vi "StringSplitter.vi"(1 "Input String":string="FPSP0RP0FS0TL0PP50%TD1000FEBL1CL0RL1FL0AL1HL1G3") -> (14 "S0":string, 15 "S1":string, 16 "S2":string, 17 "S3":string, 18 "S4":string, 19 "S5":string)   [LabVIEW 2014]
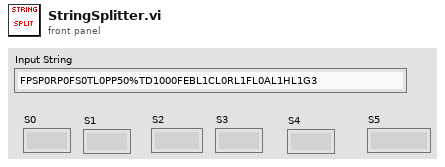
[diagram p1: front panel]
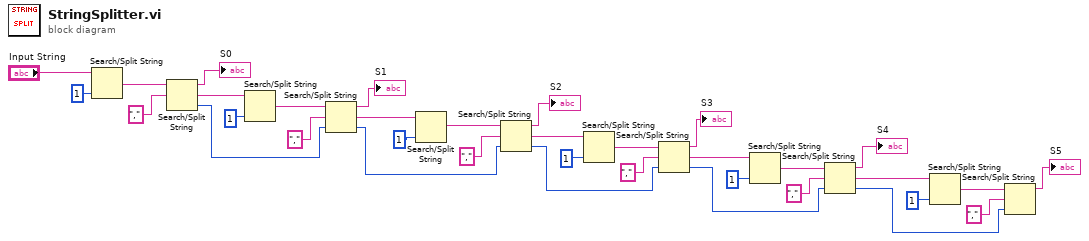
[diagram p0: block diagram]
diagram:
  n1 = Search/Split String(string="Input String", offset (0)=1) -> (match + rest of string=w33:string)  [unwired: 1 in, 2 out]
  n2 = Search/Split String(string=w33, search string/char (-)=",") -> (substring before match=→"S0":string, match + rest of string=w30:string, offset of match=w26:i32)  [unwired: 1 in]
  n3 = Search/Split String(string=w30, offset (0)=1) -> (match + rest of string=w28:string)  [unwired: 1 in, 2 out]
  n4 = Search/Split String(string=w28, search string/char (-)=",", offset (0)=w26) -> (substring before match=→"S1":string, match + rest of string=w24:string, offset of match=w21:i32)
  n5 = Search/Split String(string=w24, offset (0)=1) -> (match + rest of string=w22:string)  [unwired: 1 in, 2 out]
  n6 = Search/Split String(string=w22, search string/char (-)=",", offset (0)=w21) -> (substring before match=→"S2":string, match + rest of string=w18:string, offset of match=w13:i32)
  n7 = Search/Split String(string=w18, offset (0)=1) -> (match + rest of string=w16:string)  [unwired: 1 in, 2 out]
  n8 = Search/Split String(string=w16, search string/char (-)=",", offset (0)=w13) -> (substring before match=→"S3":string, match + rest of string=w9:string, offset of match=w8:i32)
  n9 = Search/Split String(string=w9, offset (0)=1) -> (match + rest of string=w11:string)  [unwired: 1 in, 2 out]
  n10 = Search/Split String(string=w11, search string/char (-)=",", offset (0)=w8) -> (substring before match=→"S4":string, match + rest of string=w3:string, offset of match=w2:i32)
  n11 = Search/Split String(string=w3, offset (0)=1) -> (match + rest of string=w5:string)  [unwired: 1 in, 2 out]
  n12 = Search/Split String(string=w5, search string/char (-)=",", offset (0)=w2) -> (substring before match=→"S5":string)  [unwired: 2 out]
